vi "RichToFlatni_measurementlink_sessionmanagement_v1_ReserveSessionsResponse.vi"(5 "OutputClusterType":T1, 11 "InputCluster":T8) -> (3 "OutputCluster":T1)   [LabVIEW 2020, in "Measurement Plugin Session Management Client.lvlib"]
uses:
  Measurement Plugin Session Management Client.lvlib
  ni_measurementlink_sessionmanagement_v1_ReserveSessionsResponse.ctl
  ni_measurementlink_sessionmanagement_v1_SessionInformation.ctl
  nidevice_grpc_Session.ctl
  ni_measurementlink_sessionmanagement_v1_ChannelMapping.ctl
  ni_measurementlink_sessionmanagement_v1_MultiplexerSessionInformation.ctl
  ni_measurementlink_sessionmanagement_v1_ReserveSessionsResponse_GroupMappingsEntry.ctl
  ni_measurementlink_sessionmanagement_v1_ResolvedPinsOrRelays.ctl
  ni_measurementlink_sessionmanagement_v1_ReserveSessionsResponse_Flat.ctl
  ni_measurementlink_sessionmanagement_v1_SessionInformation_Flat.ctl
  nidevice_grpc_Session_Flat.ctl
  ni_measurementlink_sessionmanagement_v1_ChannelMapping_Flat.ctl
  ni_measurementlink_sessionmanagement_v1_MultiplexerSessionInformation_Flat.ctl
  ni_measurementlink_sessionmanagement_v1_ReserveSessionsResponse_GroupMappingsEntry_Flat.ctl
  ni_measurementlink_sessionmanagement_v1_ResolvedPinsOrRelays_Flat.ctl
  RichToFlatnidevice_grpc_Session.vi
  RichToFlatni_measurementlink_sessionmanagement_v1_ChannelMapping.vi
  RichToFlatni_measurementlink_sessionmanagement_v1_ResolvedPinsOrRelays.vi
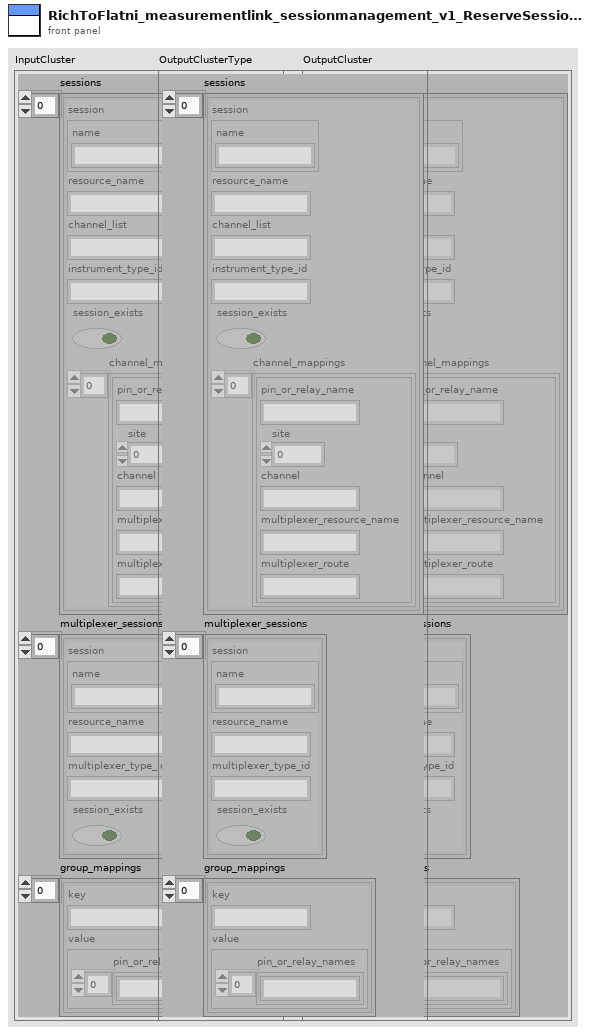
[diagram p1: front panel]
types:
  T1 = typedef "Measurement Plugin Session Management Client.lvlib/ni_measurementlink_sessionmanagement_v1_ReserveSessionsResponse_Flat.ctl" = cluster{"sessions":T2[], "multiplexer_sessions":T5[], "group_mappings":T6[]}
  T2 = typedef "Measurement Plugin Session Management Client.lvlib/ni_measurementlink_sessionmanagement_v1_SessionInformation_Flat.ctl" = cluster{"session":T3, "resource_name":string, "channel_list":string, "instrument_type_id":string, "session_exists":bool, "channel_mappings":T4[]}
  T3 = typedef "Measurement Plugin Session Management Client.lvlib/nidevice_grpc_Session_Flat.ctl" = cluster{"name":string}
  T4 = typedef "Measurement Plugin Session Management Client.lvlib/ni_measurementlink_sessionmanagement_v1_ChannelMapping_Flat.ctl" = cluster{"pin_or_relay_name":string, "site":i32, "channel":string, "multiplexer_resource_name":string, "multiplexer_route":string}
  T5 = typedef "Measurement Plugin Session Management Client.lvlib/ni_measurementlink_sessionmanagement_v1_MultiplexerSessionInformation_Flat.ctl" = cluster{"session":T3, "resource_name":string, "multiplexer_type_id":string, "session_exists":bool}
  T6 = typedef "Measurement Plugin Session Management Client.lvlib/ni_measurementlink_sessionmanagement_v1_ReserveSessionsResponse_GroupMappingsEntry_Flat.ctl" = cluster{"key":string, "value":T7}
  T7 = typedef "Measurement Plugin Session Management Client.lvlib/ni_measurementlink_sessionmanagement_v1_ResolvedPinsOrRelays_Flat.ctl" = cluster{"pin_or_relay_names":string[]}
  T8 = typedef "Measurement Plugin Session Management Client.lvlib/ni_measurementlink_sessionmanagement_v1_ReserveSessionsResponse.ctl" = cluster{"sessions":T9[], "multiplexer_sessions":T12[], "group_mappings":T13[]}
  T9 = typedef "Measurement Plugin Session Management Client.lvlib/ni_measurementlink_sessionmanagement_v1_SessionInformation.ctl" = cluster{"session":T10, "resource_name":string, "channel_list":string, "instrument_type_id":string, "session_exists":bool, "channel_mappings":T11[]}
  T10 = typedef "Measurement Plugin Session Management Client.lvlib/nidevice_grpc_Session.ctl" = cluster{"name":string}
  T11 = typedef "Measurement Plugin Session Management Client.lvlib/ni_measurementlink_sessionmanagement_v1_ChannelMapping.ctl" = cluster{"pin_or_relay_name":string, "site":i32, "channel":string, "multiplexer_resource_name":string, "multiplexer_route":string}
  T12 = typedef "Measurement Plugin Session Management Client.lvlib/ni_measurementlink_sessionmanagement_v1_MultiplexerSessionInformation.ctl" = cluster{"session":T10, "resource_name":string, "multiplexer_type_id":string, "session_exists":bool}
  T13 = typedef "Measurement Plugin Session Management Client.lvlib/ni_measurementlink_sessionmanagement_v1_ReserveSessionsResponse_GroupMappingsEntry.ctl" = cluster{"key":string, "value":T14}
  T14 = typedef "Measurement Plugin Session Management Client.lvlib/ni_measurementlink_sessionmanagement_v1_ResolvedPinsOrRelays.ctl" = cluster{"pin_or_relay_names":string[]}
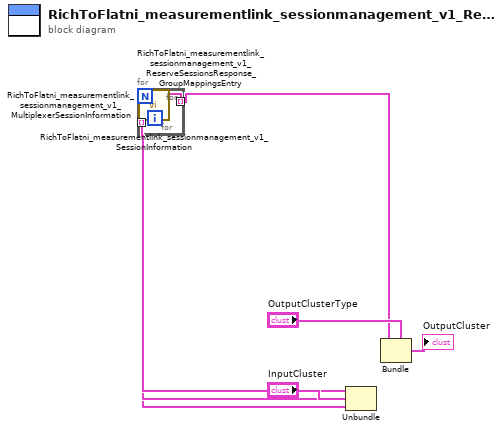
[diagram p0: block diagram]
diagram:
  n1 = Unbundle "Unbundle"("InputCluster") -> ("sessions"=w6:T9[], "multiplexer_sessions"=w4:T12[], "group_mappings"=w2:T13[])
  n2 = for {
    tunnel: w2 -> [w11] mode=indexing
    tunnel: [w10] -> w1 mode=indexing
    n3 = call "RichToFlatni_measurementlink_sessionmanagement_v1_ReserveSessionsResponse_GroupMappingsEntry.vi"("InputCluster"=w11) -> ("OutputCluster"=w10:T6)  [unwired: 10 in]
  }
  n4 = for {
    tunnel: w4 -> [w13] mode=indexing
    tunnel: [w12] -> w3 mode=indexing
    n5 = call "RichToFlatni_measurementlink_sessionmanagement_v1_MultiplexerSessionInformation.vi"("InputCluster"=w13) -> ("OutputCluster"=w12:T5)  [unwired: 10 in]
  }
  n6 = for {
    tunnel: w6 -> [w15] mode=indexing
    tunnel: [w14] -> w5 mode=indexing
    n7 = call "RichToFlatni_measurementlink_sessionmanagement_v1_SessionInformation.vi"("InputCluster"=w15) -> ("OutputCluster"=w14:T2)  [unwired: 10 in]
  }
  n8 = Bundle "Bundle"(cluster="OutputClusterType", "sessions"=w5, "multiplexer_sessions"=w3, "group_mappings"=w1) -> (→"OutputCluster":T1)
